vi "RAW DATA.vi"(8 "error in 2":errorcluster, 10 "String":string, 11 "array":path[](array[path])) -> (0 "error out 9":errorcluster)   [LabVIEW 2025]
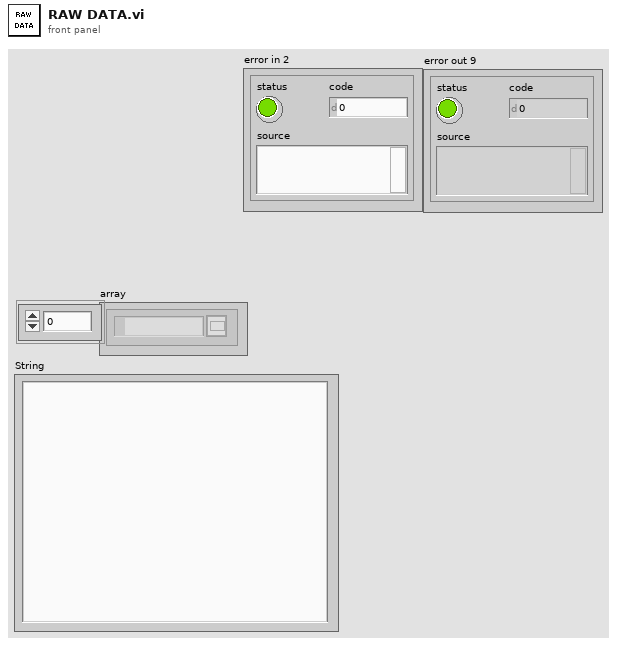
[diagram p1: front panel]
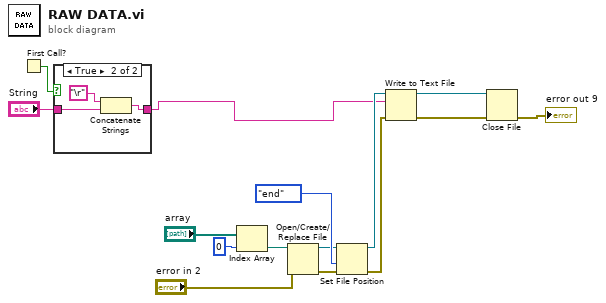
[diagram p0: block diagram]
diagram:
  n1 = First Call?() -> (First Call?: T/F=w5:bool)
  n2 = case shown="True" w5 {
    tunnel: [w16 w18] -> w1
    tunnel: "String" -> [w16 w17]
    frame False {
    }
    frame True {
      n3 = Concatenate Strings("\r", w17) -> (w18:string)
    }
  }
  n4 = Index Array(array="array", index=0 ("index (row)")) -> (element=w7:path)
  n5 = Open/Create/Replace File(file path (use dialog)=w7, error in="error in 2") -> (refnum out=w8:refnum<file>, error out=w11:errorcluster)  [unwired: 4 in, 1 out]
  n6 = Set File Position(refnum=w8, from (0:start)=enum16{"start", "end", "current"}."end", error in=w11) -> (refnum out=w9:refnum<file>, error out=w10:errorcluster)  [unwired: 1 in]
  n7 = Write to Text File(file (use dialog)=w9, text=w1, error in=w10) -> (refnum out=w13:refnum<file>, error out=w12:errorcluster)  [unwired: 1 in, 1 out]
  n8 = Close File(refnum=w13, error in=w12) -> (error out=→"error out 9":errorcluster)  [unwired: 1 out]
